vi "Untitled 1.vi"() -> ()   [LabVIEW 2020]
uses:
  <vilib>/addons/database/NI_Database_API.lvlib
  <vilib>/addons/database/_DB Variant To Data/Database Variant To Data.xnode
  <vilib>/addons/database/Connection.llb/Conn ObjectReference.ctl
panel:
  out "error out":errorcluster
  in  "error in (no error)":errorcluster
  out "connection reference out":T1
  in  "connection reference":T1
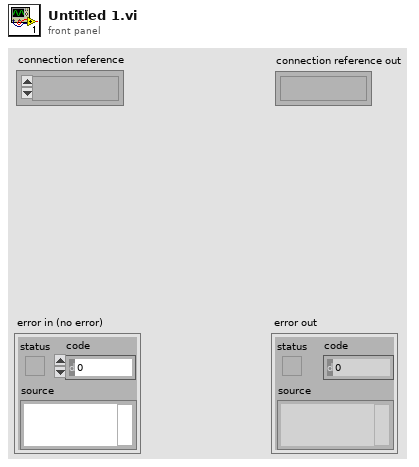
[diagram p1: front panel]
types:
  T1 = typedef "NI_Database_API.lvlib/Conn ObjectReference.ctl" = refnum<k1>
  T2 = typedef "NI_Database_API.lvlib/Conn DataMembers.ctl" = cluster{"ADODB._Connection":refnum<k7>, "recordset objects":i32, "command objects":i32}
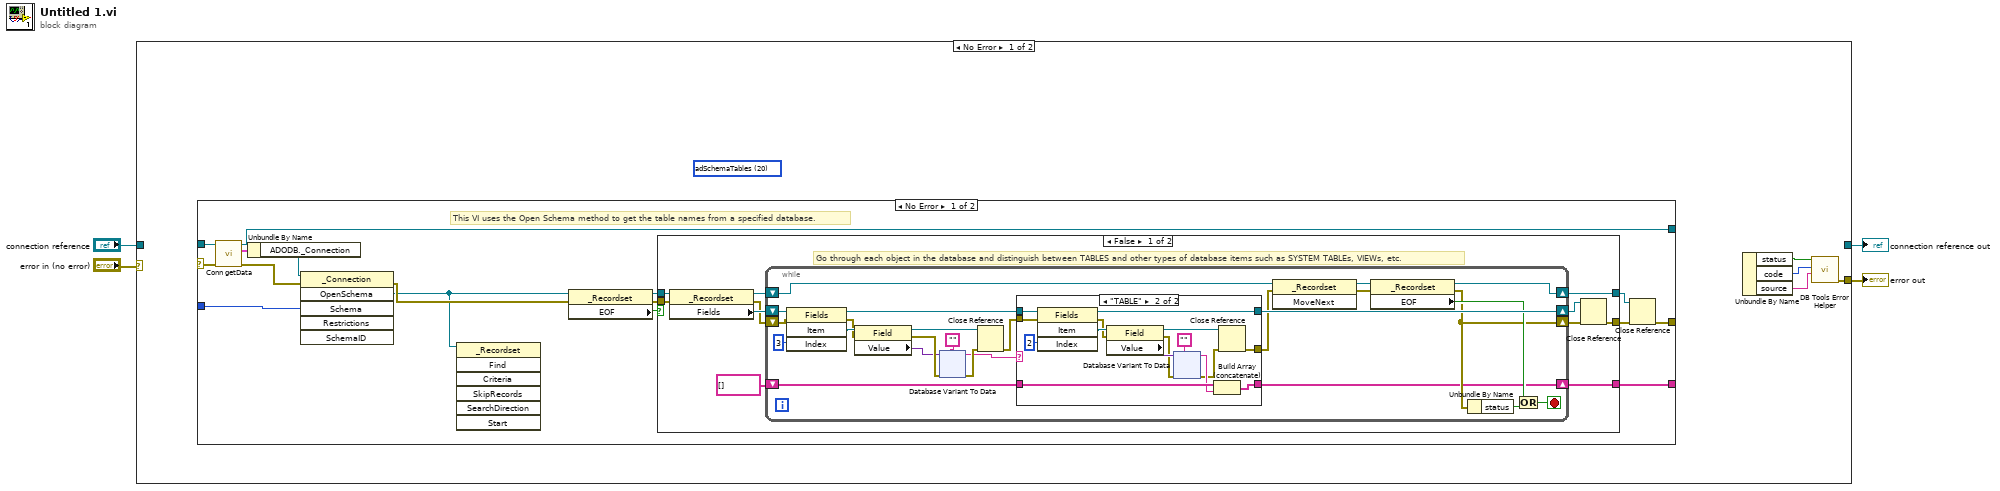
[diagram p0: block diagram]
diagram:
  n1 = case shown="No Error" "error in (no error)" {
    selector: "error in (no error)" -> [_ w148]
    tunnel: "connection reference" -> [_ w147]
    tunnel: [_ w147] -> w3
    tunnel: [w6 w148] -> w2
    frame No Error {
      (unwired) 20 items=["adSchemaProviderSpecific"=-1, "adSchemaAsserts"=0, "adSchemaCatalogs"=1, "adSchemaCharacterSets"=2, "adSchemaCollations"=3, "adSchemaColumns"=4, "adSchemaCheckConstraints"=5, "adSchemaConstraintColumnUsage"=6, "adSchemaConstraintTableUsage"=7, "adSchemaKeyColumnUsage"=8, "adSchemaReferentialContraints, adSchemaReferentialConstraints"=9, "adSchemaTableConstraints"=10, "adSchemaColumnsDomainUsage"=11, "adSchemaIndexes"=12, "adSchemaColumnPrivileges"=13, "adSchemaTablePrivileges"=14, "adSchemaUsagePrivileges"=15, "adSchemaProcedures"=16, "adSchemaSchemata"=17, "adSchemaSQLLanguages"=18, "adSchemaStatistics"=19, "adSchemaTables"=20, "adSchemaTranslations"=21, "adSchemaProviderTypes"=22, "adSchemaViews"=23, "adSchemaViewColumnUsage"=24, "adSchemaViewTableUsage"=25, "adSchemaProcedureParameters"=26, "adSchemaForeignKeys"=27, "adSchemaPrimaryKeys"=28, "adSchemaProcedureColumns"=29, "adSchemaDBInfoKeywords"=30, "adSchemaDBInfoLiterals"=31, "adSchemaCubes"=32, "adSchemaDimensions"=33, "adSchemaHierarchies"=34, "adSchemaLevels"=35, "adSchemaMeasures"=36, "adSchemaProperties"=37, "adSchemaMembers"=38, "adSchemaTrustees"=39] ("schema")
      n2 = case shown="No Error" {
        selector: _ -> [w10 w146]
        tunnel: _ -> [w23 w145]
        tunnel: _ -> [w21 _]
        tunnel: [w19 w145] -> _
        tunnel: [w18 _] -> _
        tunnel: [w16 w146] -> _
        frame No Error {
          # "This VI uses the Open Schema method to get the table names from a specified database."
          n3 = call <vilib>:"Conn getData.vi"("error in (no error)"=w10, "connection reference"=w23) -> ("error out"=w20:errorcluster, "data"=w24:T2, "connection reference out"=w19:T1)  [unwired: 2 in, 1 out]
          n4 = Unbundle By Name(w24) -> ("ADODB._Connection"=w22:refnum<k7>)
          n5 = invoke class="_Connection" method="OpenSchema"(reference=w22, error in=w20, "Schema"=w21) -> (error out=w13:errorcluster, "OpenSchema"=w9:refnum<k7>)  [unwired: 3 in, 4 out]
          n6 = invoke class="_Recordset" method="Find"(reference=w9) -> ()  [unwired: 6 in, 7 out]
          n7 = property class="_Recordset"(reference=w9, error in=w13) -> (reference out=w14:refnum<k7>, error out=w12:errorcluster, "EOF"=w11:bool)
          n8 = case shown="False" w11 {
            tunnel: [w32 _] -> w18
            tunnel: [w29 w143] -> w17
            tunnel: [w27 w144] -> w15
            tunnel: w14 -> [w26 w144]
            tunnel: w12 -> [w25 w143]
            frame False {
              # "Go through each object in the database and distinguish between TABLES and other types of database items such as SYSTEM TABLEs, VIEWs, etc."
              n9 = property class="_Recordset"(reference=w26, error in=w25) -> (reference out=w35:refnum<k7>, error out=w33:errorcluster, "Fields"=w34:refnum<k7>)
              n10 = while {
                shift-right: [w52] -> w28
                shift-left: w34 -> [w60]
                shift-right: [w46] -> w30
                shift-left: w33 -> [w58]
                shift-right: [w55] -> w27
                shift-left: w35 -> [w37]
                shift-right: [w43] -> w32
                shift-left: string[] [] -> [w44]
                stop <- w59 stop-if-true
                n11 = invoke class="Fields" method="Item"(reference=w60, error in=w58, "Index"=3) -> (reference out=w53:refnum<k7>, error out=w36:errorcluster, "Item"=w51:refnum<k7>)  [unwired: 1 in, 1 out]
                n12 = property class="Field"(reference=w51, error in=w36) -> (reference out=w41:refnum<k7>, error out=w49:errorcluster, "Value"=w42:variant)
                n13 = xnode "Database Variant To Data"("database variant"=w42, "error in"=w49, "type"="") -> ("data"=w38:string, "error out"=w40:errorcluster)
                n14 = Close Reference(reference=w41, error in (no error)=w40) -> (error out=w39:errorcluster)
                n15 = case shown="\"TABLE\"" w38 {
                  tunnel: [w94 w103] -> w43
                  tunnel: w53 -> [w95 w109]
                  tunnel: [w95 w107] -> w52
                  tunnel: [w93 w97] -> w45
                  tunnel: w44 -> [w94 w104]
                  tunnel: w39 -> [w93 w99]
                  frame Default {
                  }
                  frame "TABLE" {
                    n16 = invoke class="Fields" method="Item"(reference=w109, error in=w99, "Index"=2) -> (reference out=w107:refnum<k7>, error out=w106:errorcluster, "Item"=w108:refnum<k7>)  [unwired: 1 in, 1 out]
                    n17 = property class="Field"(reference=w108, error in=w106) -> (reference out=w96:refnum<k7>, error out=w100:errorcluster, "Value"=w101:variant)
                    n18 = xnode "Database Variant To Data"("database variant"=w101, "error in"=w100, "type"="") -> ("data"=w102:string, "error out"=w98:errorcluster)
                    n19 = Build Array (concatenate)(w104, w102) -> (w103:string[])
                    n20 = Close Reference(reference=w96, error in (no error)=w98) -> (error out=w97:errorcluster)
                  }
                }
                n21 = invoke class="_Recordset" method="MoveNext"(reference=w37, error in=w45) -> (reference out=w57:refnum<k7>, error out=w56:errorcluster)  [unwired: 1 in, 1 out]
                n22 = property class="_Recordset"(reference=w57, error in=w56) -> (reference out=w55:refnum<k7>, error out=w46:errorcluster, "EOF"=w47:bool)
                n23 = Unbundle By Name(w46) -> ("status"=w54:bool)
                n24 = Or(x=w47, y=w54) -> (x .or. y?=w59:bool)
              }
              n25 = Close Reference(reference=w28, error in (no error)=w30) -> (error out=w29:errorcluster)
            }
            frame True {
              # "No objects in the database."
            }
          }
          n26 = Close Reference(reference=w15, error in (no error)=w17) -> (error out=w16:errorcluster)
        }
        frame Error {
        }
      }
      n27 = Unbundle By Name() -> ("status"=w7:bool, "code"=w5:i32, "source"=w8:string)  [unwired: 1 in]
      n28 = call <vilib>:"DB Tools Error Helper.vi"("source"=w8, "code"=w5, "status"=w7) -> ("error out"=w6:errorcluster)  [unwired: 1 in, 7 out]
    }
    frame Error {
    }
  }
  "connection reference out" <- w3
  "error out" <- w2
